vi "Add Calculate Channel_Peak and Valley_Peak and Valley.vi"(7 "SysDef Ref":T1, 8 "error in (error out)":errorcluster, 9 "Peak and Valley Settings":T2={"Name"="", "Description"="", "Channel to Analyze Node Path"="", "Channel to Valley Node Path"="", "Channel to Offset Node Path"="", "Reset"=100, "Hysteresis"=0.2, "Alias Name"=""}, 11 "Calculated Channels Ref":refnum<k24>) -> (0 "error out":errorcluster, 3 "Calculated Channels Ref Out":refnum<k24>)   [LabVIEW 2019, in "Simple SysDef API.lvlib"]
uses:
  <userlib>/SimpleSysDef/Simple SysDef API.lvlib
  NationalInstruments.VeriStand.SystemDefinitionAPI
  <userlib>/SimpleSysDef/_SubVIs/Add Calculate Channel_Peak and Valley_Settings.ctl
  <userlib>/SimpleSysDef/_SubVIs/System Definition Reference.ctl
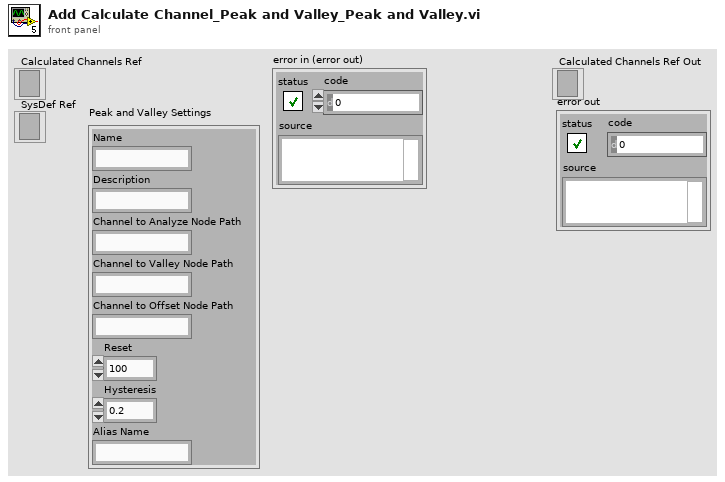
[diagram p1: front panel]
types:
  T1 = typedef "Simple SysDef API.lvlib/System Definition Reference.ctl" = refnum<k24>
  T2 = typedef "Simple SysDef API.lvlib/Add Calculate Channel_Peak and Valley_Settings.ctl" = cluster{"Name":string, "Description":string, "Channel to Analyze Node Path":string, "Channel to Valley Node Path":string, "Channel to Offset Node Path":string, "Reset":u32, "Hysteresis":dbl, "Alias Name":string}
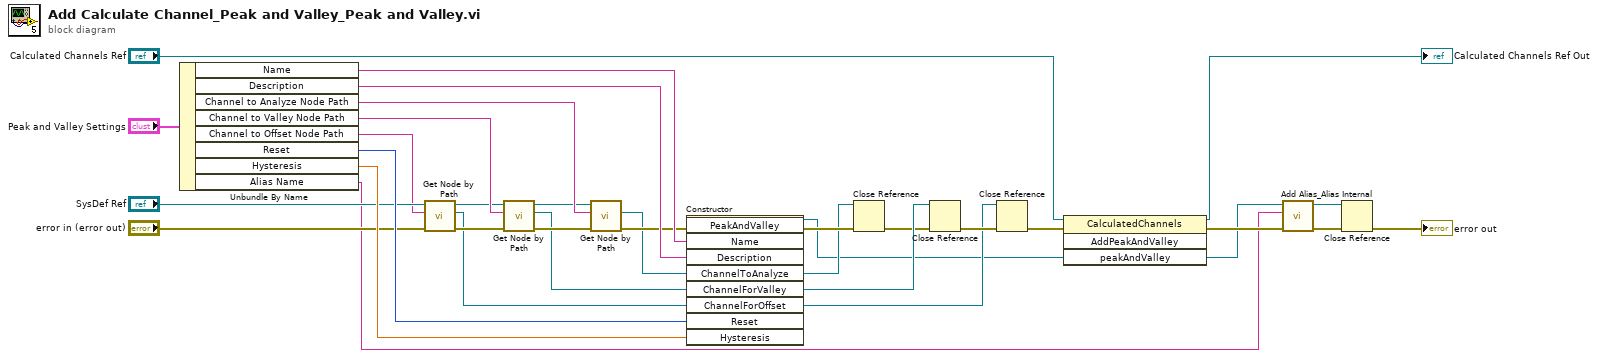
[diagram p0: block diagram]
diagram:
  n1 = Unbundle By Name("Peak and Valley Settings") -> ("Name"=w26:string, "Description"=w25:string, "Channel to Analyze Node Path"=w20:string, "Channel to Valley Node Path"=w24:string, "Channel to Offset Node Path"=w12:string, "Reset"=w18:u32, "Hysteresis"=w17:dbl, "Alias Name"=w1:string)
  n2 = call <userlib>:"Get Node by Path.vi"("error in (no error)"="error in (error out)", "System Definition Node Path"=w12, "SysDef Ref"="SysDef Ref") -> ("error out"=w15:errorcluster, "Node Ref"=w7:refnum<k24>, "SysDef Ref Out"=w16:T1)  [unwired: 6 in]
  n3 = call <userlib>:"Get Node by Path.vi"("error in (no error)"=w15, "System Definition Node Path"=w24, "SysDef Ref"=w16) -> ("error out"=w22:errorcluster, "Node Ref"=w21:refnum<k24>, "SysDef Ref Out"=w19:T1)  [unwired: 6 in]
  n4 = call <userlib>:"Get Node by Path.vi"("error in (no error)"=w22, "System Definition Node Path"=w20, "SysDef Ref"=w19) -> ("error out"=w23:errorcluster, "Node Ref"=w6:refnum<k24>)  [unwired: 6 in, 1 out]
  n5 = constructor class="PeakAndValley"(error in=w23, "Name"=w26, "Description"=w25, "ChannelToAnalyze"=w6, "ChannelForValley"=w21, "ChannelForOffset"=w7, "Reset"=w18, "Hysteresis"=w17) -> (reference out=w3:refnum<k24>, error out=w11:errorcluster)  [unwired: 2 in, 8 out]
  n6 = Close Reference(reference=w6, error in (no error)=w11) -> (error out=w10:errorcluster)
  n7 = Close Reference(reference=w21, error in (no error)=w10) -> (error out=w9:errorcluster)
  n8 = Close Reference(reference=w7, error in (no error)=w9) -> (error out=w8:errorcluster)
  n9 = invoke class="CalculatedChannels" method="AddPeakAndValley"(reference="Calculated Channels Ref", error in=w8, "peakAndValley"=w3) -> (reference out=→"Calculated Channels Ref Out":refnum<k24>, error out=w5:errorcluster)  [unwired: 1 in, 2 out]
  n10 = call <userlib>:"Add Alias_Alias Internal.vi"("error in (no error)"=w5, "Name"=w1, "Base Node"=w3) -> ("error out"=w4:errorcluster, "Base Node out"=w2:refnum<k24>)  [unwired: 7 in]
  n11 = Close Reference(reference=w2, error in (no error)=w4) -> (error out=→"error out":errorcluster)
